vi "LBCB Units DAO.vi"(7 "refnum in":T1, 8 "error in (no error)":errorcluster, 9 "Index":i32, 10 "Unit Labels In":string[](array[string]), 11 "Persistent DAO Actions":T2) -> (0 "error out":errorcluster, 1 "DOF Type":string[](array[string])=["Actuator.Displacement", "Actuator.Force", "Cartesian.Translation", "Cartesian.Rotation", "Cartesian.Force", "Cartesian.Moment"], 2 "Unit Labels Out":string[](array[string]), 3 "Unit":string, 4 "refnum out":T1)   [LabVIEW 2013]
uses:
  Metadata/Persistant DAO Actions.ctl
  <vilib>/Utility/config.llb/Config Data RefNum.ctl
  <vilib>/Utility/config.llb/Read Key (String).vi
  <vilib>/Utility/config.llb/Write Key (String).vi
  <vilib>/Utility/config.llb/NI_LVConfig.lvlib
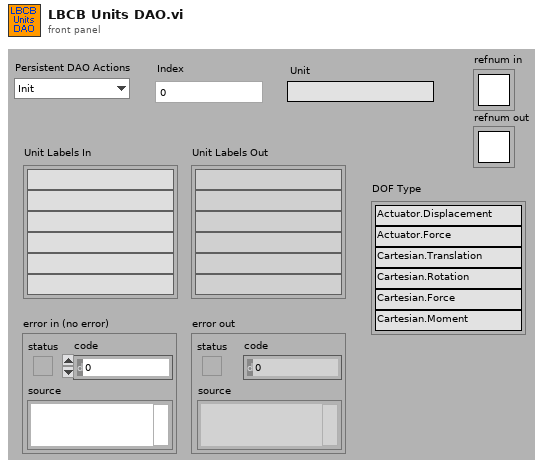
[diagram p1: front panel]
types:
  T1 = typedef "NI_LVConfig.lvlib/Config Data RefNum.ctl" = refnum<k1>
  T2 = typedef "Persistant DAO Actions.ctl" = enum16{"Init", "Get", "Set", "Load", "Save"}
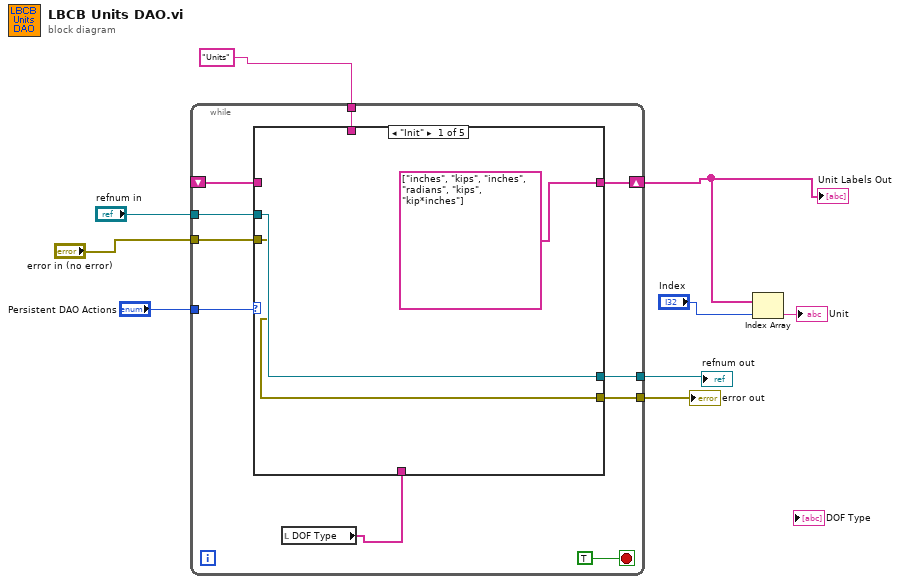
[diagram p0: block diagram]
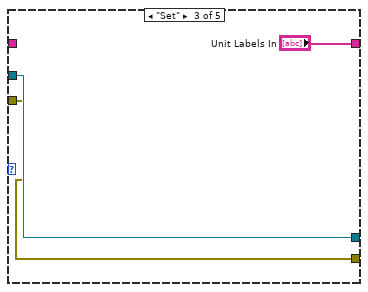
[diagram p3: hidden frame]
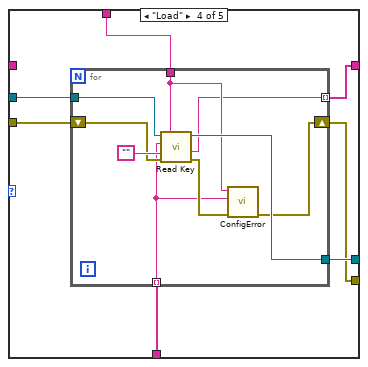
[diagram p4: hidden frame]
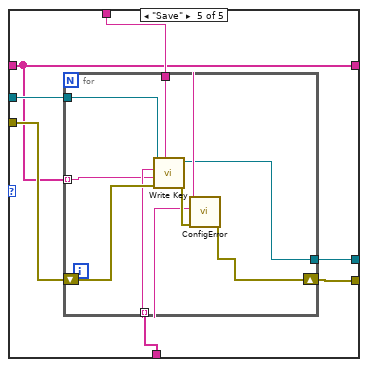
[diagram p5: hidden frame]
diagram:
  n1 = while {
    tunnel: "Persistent DAO Actions" -> [w18]
    shift-right: [w17] -> w3
    shift-left: _ -> [w16]
    tunnel: "Units" ("section") -> [w15]
    tunnel: "refnum in" -> [w14]
    tunnel: "error in (no error)" -> [w13]
    tunnel: [w12] -> w6
    tunnel: [w11] -> w5
    stop <- TRUE stop-if-true
    n2 = local read "DOF Type"() -> (w10:string[])
    n3 = case shown="\"Init\"" w18 {
      tunnel: [string[] ["inches", "kips", "inches", "radians", "kips", "kip*inches"] ("DOF Type") w25 "Unit Labels In" w29 w47] -> w17
      tunnel: w16 -> [_ w25 _ _ w47]
      tunnel: w15 -> [_ _ _ w32 w49]
      tunnel: w14 -> [w22 w24 w27 w33 w51]
      tunnel: w13 -> [w21 w23 w26 w30 w50]
      tunnel: w10 -> [_ _ _ w31 w48]
      tunnel: [w22 w24 w27 w35 w45] -> w12
      tunnel: [w21 w23 w26 w34 w46] -> w11
      frame "Init" {
      }
      frame "Get" {
      }
      frame "Set" {
      }
      frame "Load" {
        n4 = for {
          tunnel: [w44] -> w35
          tunnel: w33 -> [w41]
          tunnel: w32 -> [w37]
          tunnel: w31 -> [w38] mode=indexing
          shift-right: [w42] -> w34
          shift-left: w30 -> [w39]
          tunnel: [w36] -> w29 mode=indexing
          n5 = call-poly <vilib>:"Read Key.vi"("section"=w37, "error in (no error)"=w39, "default value"="", "key"=w38, "refnum"=w41) -> ("error out"=w43:errorcluster, "value"=w36:string, "refnum out"=w44:T1)  [unwired: 1 in, 3 out]
          n6 = call "ConfigError.vi"("error in (no error)"=w43, "Key"=w38, "Section"=w37) -> ("error out"=w42:errorcluster)  [unwired: 8 out]
        }
      }
      frame "Save" {
        n7 = for {
          tunnel: w51 -> [w59]
          tunnel: w49 -> [w56]
          tunnel: w48 -> [w55] mode=indexing
          tunnel: w47 -> [w54] mode=indexing
          tunnel: [w52] -> w45
          shift-right: [w53] -> w46
          shift-left: w50 -> [w58]
          n8 = call-poly <vilib>:"Write Key.vi"("section"=w56, "error in (no error)"=w58, "value"=w54, "key"=w55, "refnum"=w59) -> ("error out"=w57:errorcluster, "refnum out"=w52:T1)  [unwired: 1 in, 4 out]
          n9 = call "ConfigError.vi"("error in (no error)"=w57, "Key"=w55, "Section"=w56) -> ("error out"=w53:errorcluster)  [unwired: 8 out]
        }
      }
    }
  }
  "error out" <- w5
  "refnum out" <- w6
  "Unit Labels Out" <- w3
  n10 = Index Array(array=w3, index="Index") -> (element=→"Unit":string)
